vi "main.vi"() -> ()   [LabVIEW 2014]
uses:
  <vilib>/picture/3D Picture Control/Object/Create Object (drawable).vi
  <vilib>/picture/3D Picture Control/Object/Add Object (reference).vi
  <vilib>/Instr/_visa.llb/VISA Configure Serial Port (Instr).vi
  <vilib>/picture/3D Picture Control/NI_3D Picture Control.lvlib
panel:
  out "AcceZ":i32
  out "AcceY":i32
  out "加速度":cluster{dbl, dbl, dbl}(graph)
  out "AcceX":i32
  out "HEANDING":i32
  out "BANK":i32
  out "PITCH":i32
  in  "停止":bool
  in  "打开":bool caption="stop"
  in  "校验位：":u16(ring) items=["  无校验", "  奇校验", "  偶校验"]
  in  "波特率：":u16(ring)=11 items=["   300", "   600", "   1200", "   2400", "   4800   ", "   9600", "   19200", "   38400", "   43000", "   56000", "   57600", "   115200"]
  in  "通讯口：":u16(ring) items=["   com1", "   com2", "   com3", "   com4", "   com5"]
  out "姿态":cluster{dbl, dbl, dbl}(graph) caption="波形图表"
  in  "上下移动":dbl(slide) scale=-10.0..10.0
  in  "左右移动":dbl(slide) scale=-10.0..10.0
  in  "前后移动":dbl(slide) scale=-10.0..10.0
  in  "缩放":dbl(knob)=2.2771854734286614 scale=0.0..10.0
  out "三维图片":refnum<vi>(3d-picture)
  out "工作指示灯":bool
  # "----pxc"
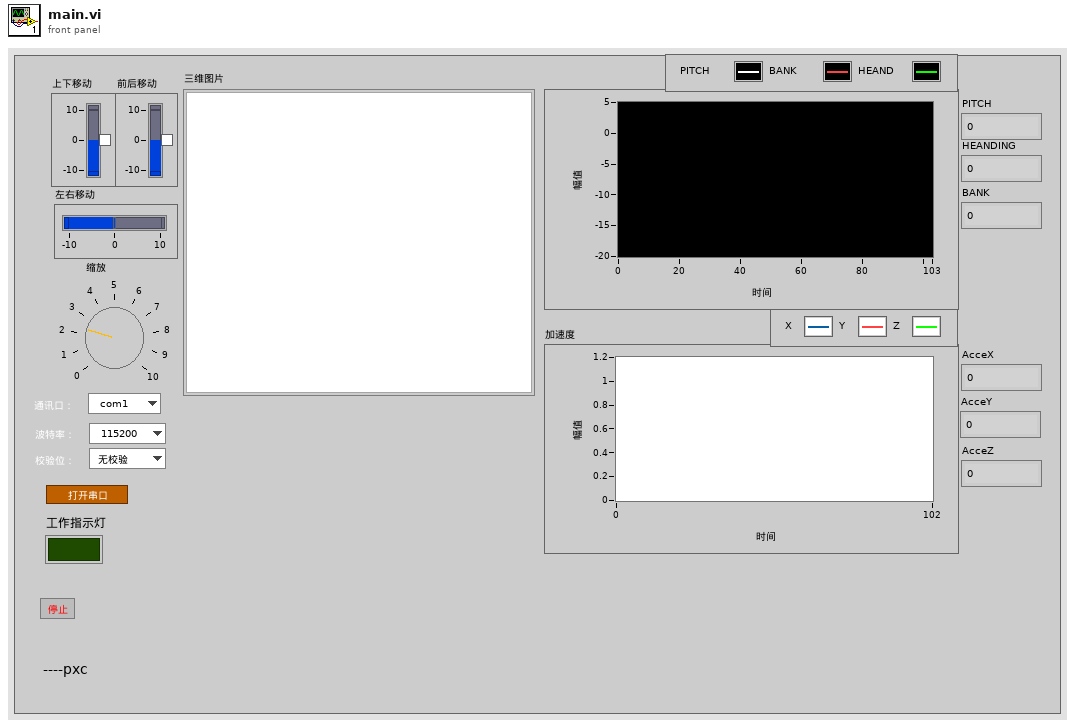
[diagram p1: front panel]
types:
  T1 = cluster{"PITCH":i32, "BANK":i32, "HEANDING":i32, "T":i32}
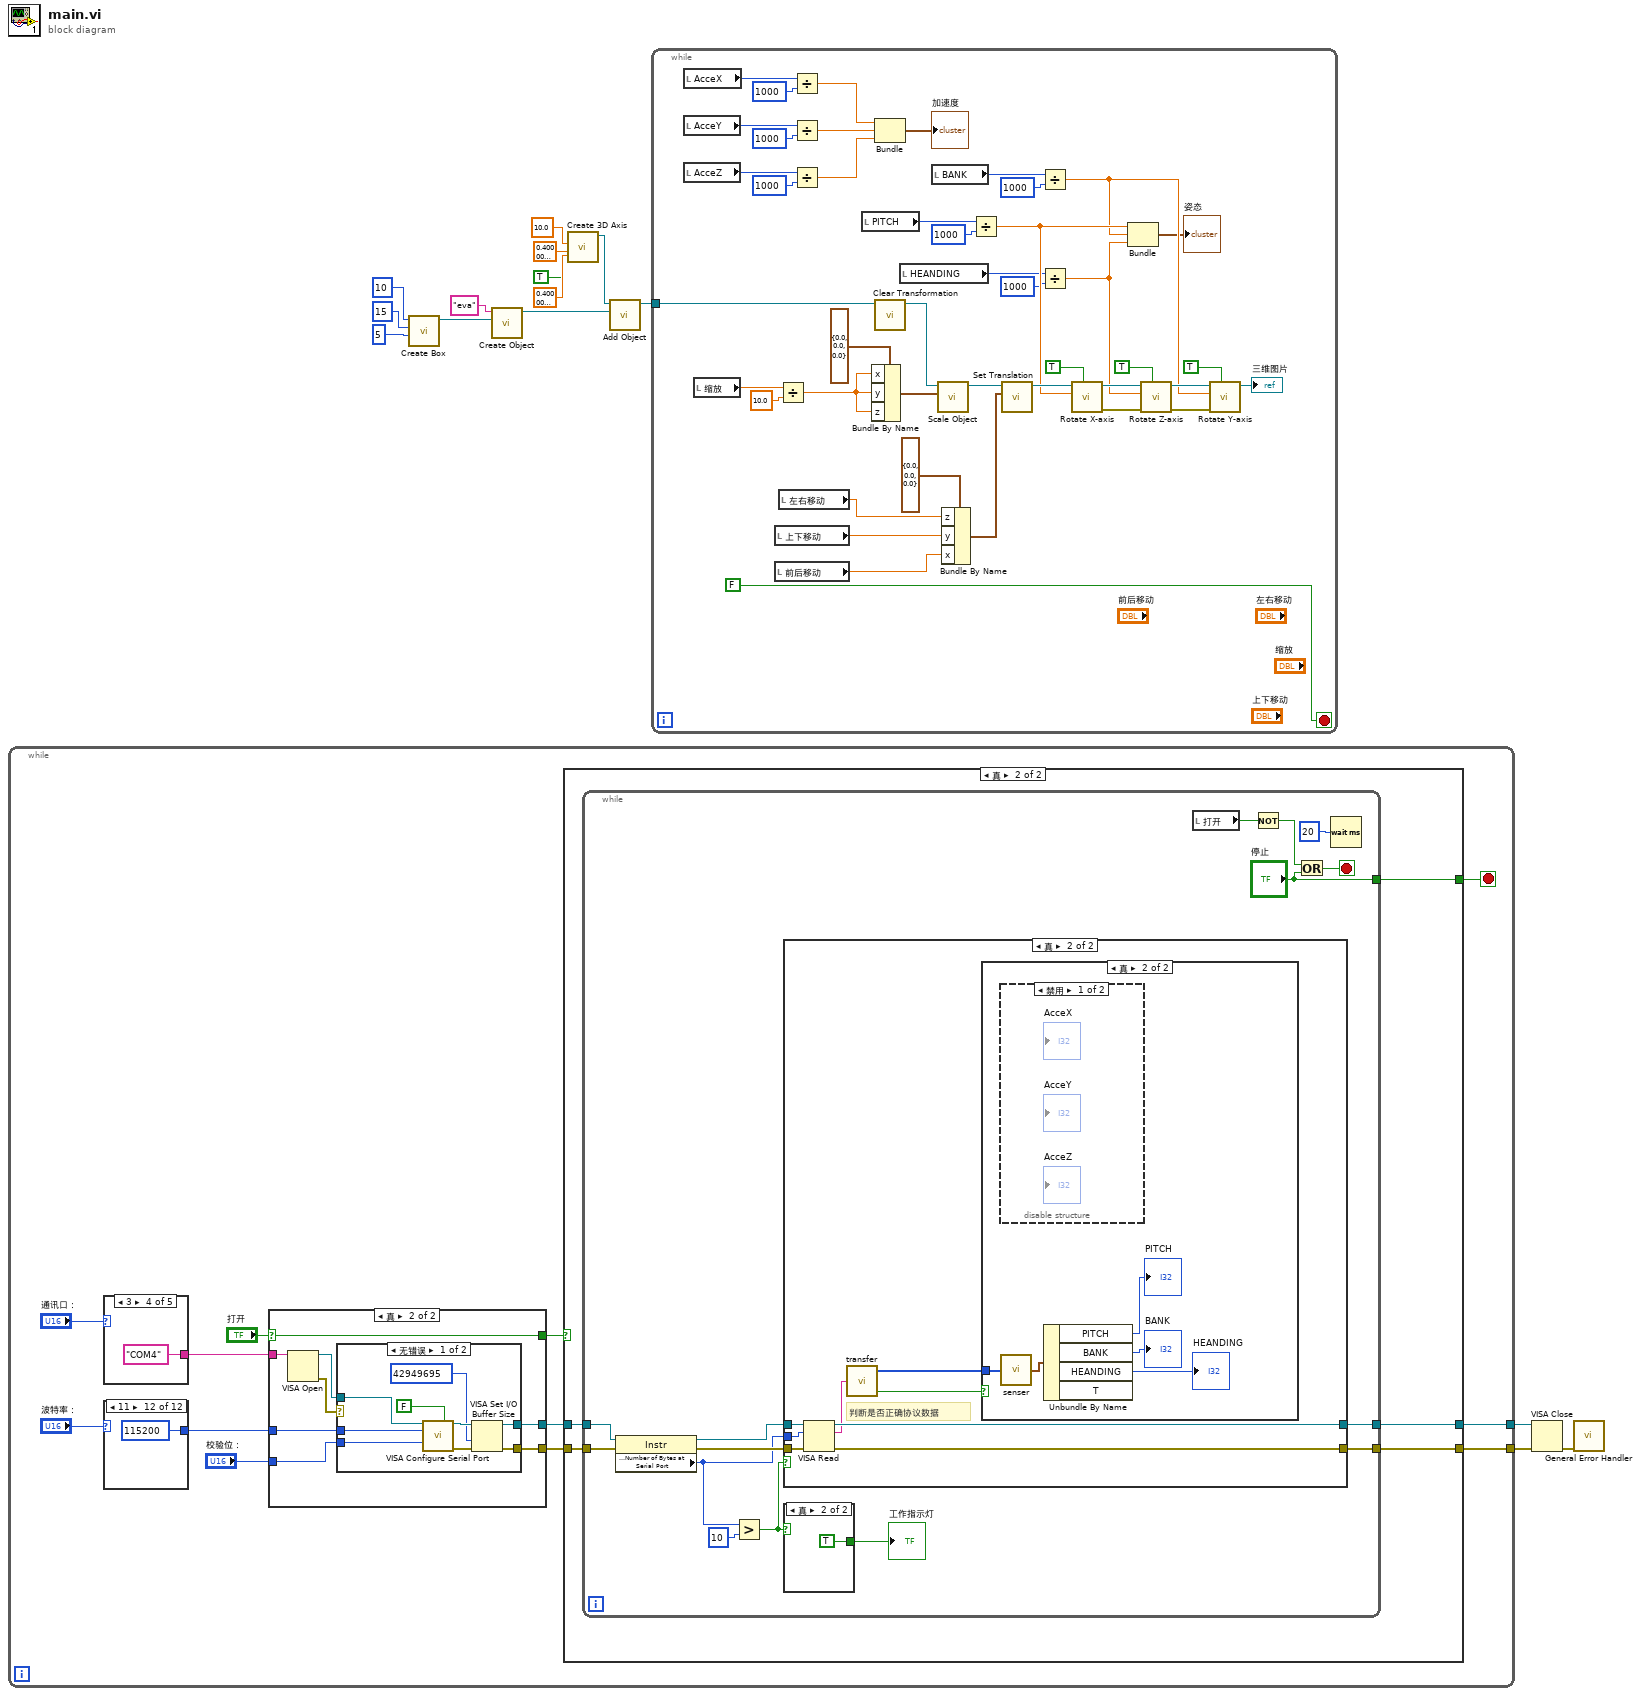
[diagram p0: block diagram]
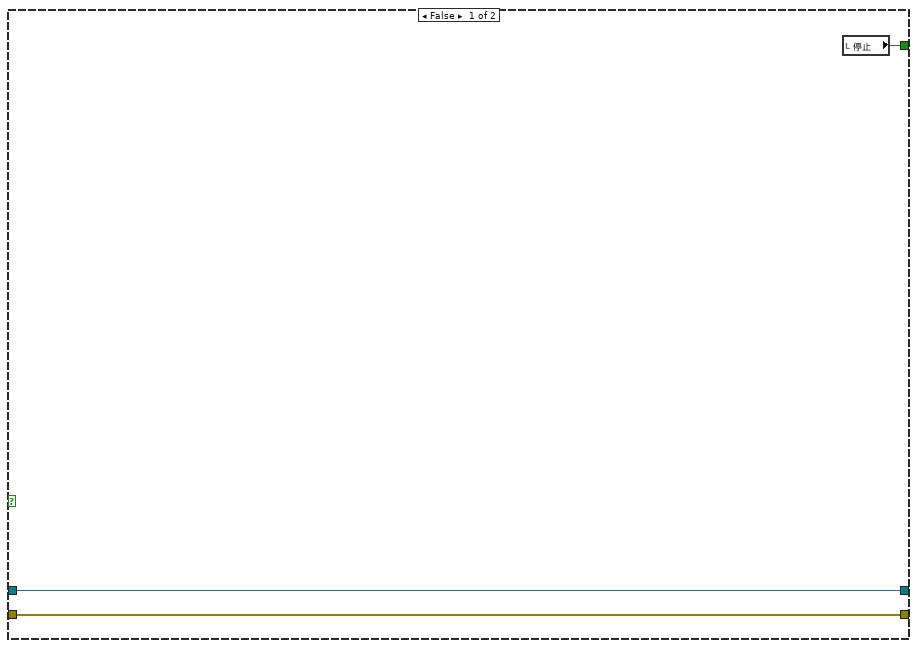
[diagram p2: hidden frame]
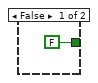
[diagram p6: hidden frame]
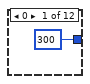
[diagram p7: hidden frame]
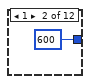
[diagram p8: hidden frame]
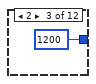
[diagram p9: hidden frame]
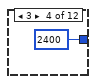
[diagram p10: hidden frame]
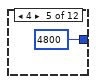
[diagram p11: hidden frame]
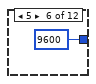
[diagram p12: hidden frame]
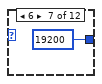
[diagram p13: hidden frame]
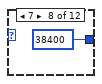
[diagram p14: hidden frame]
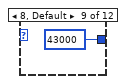
[diagram p15: hidden frame]
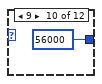
[diagram p16: hidden frame]
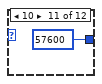
[diagram p17: hidden frame]
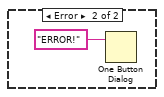
[diagram p19: hidden frame]
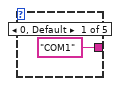
[diagram p20: hidden frame]
diagram:
  n1 = while {
    tunnel: [w26] -> w15
    tunnel: [w25] -> w14
    stop <- w17 stop-if-true
    n2 = case shown="3" "通讯口：" {
      tunnel: ["COM1" "COM2" "COM3" "COM4" "COM5"] -> w21
      frame 0, Default {
      }
      frame 1 {
      }
      frame 2 {
      }
      frame 3 {
      }
      frame 4 {
      }
    }
    n3 = case shown="11" "波特率：" {
      tunnel: [300 600 1200 2400 4800 9600 19200 38400 43000 56000 57600 115200] -> w18
      frame 0 {
      }
      frame 1 {
      }
      frame 2 {
      }
      frame 3 {
      }
      frame 4 {
      }
      frame 5 {
      }
      frame 6 {
      }
      frame 7 {
      }
      frame 8, Default {
      }
      frame 9 {
      }
      frame 10 {
      }
      frame 11 {
      }
    }
    n4 = case shown="真" "打开" {
      selector: "打开" -> [w80 w88]
      tunnel: w18 -> [_ w84]
      tunnel: [w80 w88] -> w16
      tunnel: [_ w82] -> w24
      tunnel: [_ w81] -> w27
      tunnel: w21 -> [_ w87]
      tunnel: "校验位：" -> [_ w83]
      frame False {
      }
      frame True {
        n5 = VISA Open(VISA resource name=w87) -> (VISA resource name=w85:refnum<visa-resource-name>, error out=w86:errorcluster)  [unwired: 4 in]
        n6 = case shown="无错误" w86 {
          tunnel: w85 -> [w97 _]
          tunnel: w84 -> [w96 _]
          tunnel: w83 -> [w95 _]
          tunnel: [w91 _] -> w82
          tunnel: [w92 _] -> w81
          frame No Error {
            n7 = call-poly "VISA Configure Serial Port"("VISA resource name"=w97, "Enable Termination\nChar (T)"=FALSE, "baud rate (9600)"=w96, "parity (0:none)"=w95) -> ("VISA resource name out"=w94:refnum<visa-resource-name>, "error out"=w93:errorcluster)  [unwired: 10 in]
            n8 = VISA Set I/O Buffer Size(VISA resource name=w94, size (4096)=u32 42949695 ("大小(4096)"), error in (no error)=w93) -> (VISA resource name out=w91:refnum<visa-resource-name>, error out=w92:errorcluster)  [unwired: 1 in]
          }
          frame Error {
            n9 = One Button Dialog(message="ERROR!" ("消息")) -> ()  [unwired: 1 in, 1 out]
          }
        }
      }
    }
    n10 = case shown="真" w16 {
      tunnel: w27 -> [w28 w35]
      tunnel: [w29 w34] -> w26
      tunnel: [w28 w33] -> w25
      tunnel: w24 -> [w29 w32]
      tunnel: [w30 w31] -> w17
      frame False {
        n11 = local read "停止"() -> (w30:bool)
      }
      frame True {
        n12 = while {
          tunnel: w32 -> [w42]
          tunnel: w35 -> [w41]
          tunnel: [w50] -> w34
          tunnel: [w49] -> w33
          tunnel: ["停止"] -> w31
          stop <- w46 stop-if-true
          n13 = property class="Instr"(reference=w42, error in=w41) -> (reference out=w39:refnum<visa-resource-name>, error out=w38:errorcluster, "Serial Settings:Number of Bytes at Serial Port"=w37:u32)
          n14 = Greater?(x=w37, y=u32 10) -> (0:w47:bool)
          n15 = case shown="真" w47 {
            tunnel: [w51 w54] -> w49
            tunnel: w39 -> [w52 w60]
            tunnel: w38 -> [w51 w55]
            tunnel: [w52 w59] -> w50
            tunnel: w37 -> [_ w58]
            frame False {
            }
            frame True {
              # "判断是否正确协议数据"
              n16 = VISA Read(VISA resource name=w60, byte count=w58, error in (no error)=w55) -> (VISA resource name out=w59:refnum<visa-resource-name>, read buffer=w57:string, error out=w54:errorcluster)  [unwired: 1 out]
              n17 = call "transfer.vi"("输入"=w57) -> ("待处理数据输出"=w56:u8[], "接收输出"=w53:bool)  [unwired: 1 out]
              n18 = case shown="真" w53 {
                tunnel: w56 -> [_ w65]
                frame False {
                }
                frame True {
                  n19 = disable-structure shown="禁用" {
                    frame Disabled {
                    }
                    frame Enabled {
                    }
                  }
                  n20 = call "senser.vi"("待处理数据"=w65) -> ("输出簇"=w64:T1)
                  n21 = Unbundle By Name(w64) -> ("PITCH"=→"PITCH":i32, "BANK"=→"BANK":i32, "HEANDING"=→"HEANDING":i32)  [unwired: 1 out]
                }
              }
            }
          }
          n22 = case shown="真" w47 {
            tunnel: [FALSE ("工作指示灯") TRUE ("工作指示灯")] -> w48
            frame False {
            }
            frame True {
            }
          }
          "工作指示灯" <- w48
          n23 = local read "打开"() -> (w44:bool)
          n24 = Not(x=w44) -> (.not. x?=w45:bool)
          n25 = Or(x=w45, y="停止") -> (x .or. y?=w46:bool)
          n26 = Wait (ms)(milliseconds to wait=u32 20 ("等待时间（毫秒）")) -> ()  [unwired: 1 out]
        }
      }
    }
  }
  n27 = call <vilib>:"Create Box.vi"("Length Z"=5, "Length Y"=15, "Length X"=10) -> ("New Box Refnum"=w6:refnum<vi>)  [unwired: 7 in, 1 out]
  n28 = call-poly <vilib>:"Create Object.vi"("Geometry"=w6, "Name"="eva") -> ("Scene:New Object"=w7:refnum<vi>)  [unwired: 8 in, 1 out]
  n29 = call <vilib>:"Create 3D Axis.vi"("Character Size"=sgl 0.4, "Axis label?"=TRUE, "Radius"=sgl 0.4, "Length"=sgl 10.0) -> ("New Object Refnum"=w12:refnum<vi>)  [unwired: 6 in, 1 out]
  n30 = call-poly <vilib>:"Add Object.vi"("New Object In"=w7, "Scene Object In"=w12) -> ("Scene Object Out"=w1:refnum<vi>)  [unwired: 7 in, 2 out]
  n31 = while {
    tunnel: w1 -> [w105]
    stop <- FALSE stop-if-true
    n32 = local read "AcceX"() -> (w115:i32)
    n33 = local read "AcceY"() -> (w113:i32)
    n34 = local read "AcceZ"() -> (w111:i32)
    n35 = local read "缩放"() -> (w138:dbl)
    n36 = local read "上下移动"() -> (w136:dbl)
    n37 = local read "前后移动"() -> (w135:dbl)
    n38 = Divide(x=w138, y=10.0) -> (x/y=w142:dbl)
    n39 = local read "左右移动"() -> (w137:dbl)
    n40 = Divide(x=w115, y=1000) -> (x/y=w109:dbl)
    n41 = Divide(x=w113, y=1000) -> (x/y=w108:dbl)
    n42 = Divide(x=w111, y=1000) -> (x/y=w107:dbl)
    n43 = local read "PITCH"() -> (w121:i32)
    n44 = Bundle By Name(cluster=cluster{"x":dbl, "y":dbl, "z":dbl} {"x"=0.0, "y"=0.0, "z"=0.0}, "x"=w142, "y"=w142, "z"=w142) -> (w144:cluster{"x":dbl, "y":dbl, "z":dbl})
    n45 = Bundle(w109, w108, w107) -> (→"加速度":cluster{dbl, dbl, dbl})  [unwired: 1 in]
    n46 = call <vilib>:"Clear Transformation.vi"("Object Refnum In"=w105) -> ("Object Refnum Out"=w146:refnum<vi>)  [unwired: 9 in, 1 out]
    n47 = local read "HEANDING"() -> (w117:i32)
    n48 = local read "BANK"() -> (w122:i32)
    n49 = call <vilib>:"Scale Object.vi"("Scale"=w144, "Scene.Object In"=w146) -> ("Scene.Object Out"=w145:refnum<vi>)  [unwired: 8 in, 1 out]
    n50 = Bundle By Name(cluster=cluster{"x":dbl, "y":dbl, "z":dbl} {"x"=0.0, "y"=0.0, "z"=0.0}, "z"=w137, "y"=w136, "x"=w135) -> (w141:cluster{"x":dbl, "y":dbl, "z":dbl})
    n51 = Divide(x=w121, y=1000) -> (x/y=w120:dbl)
    n52 = call <vilib>:"Set Translation.vi"("Translation"=w141, "Scene Object"=w145) -> ("Translated Object"=w132:refnum<vi>)  [unwired: 8 in, 1 out]
    n53 = Divide(x=w122, y=1000) -> (x/y=w119:dbl)
    n54 = Divide(x=w117, y=1000) -> (x/y=w123:dbl)
    n55 = call <vilib>:"Rotate X-axis.vi"("Relative?"=TRUE, "angle"=w120, "Scene Object In"=w132) -> ("error out"=w131:errorcluster, "Scene Object Out"=w130:refnum<vi>)  [unwired: 7 in]
    n56 = Bundle(w120, w119, w123) -> (→"姿态":cluster{dbl, dbl, dbl})  [unwired: 1 in]
    n57 = call <vilib>:"Rotate Z-axis.vi"("Relative?"=TRUE, "error in (no error)"=w131, "angle"=w123, "Scene Object In"=w130) -> ("error out"=w127:errorcluster, "Scene Object Out"=w126:refnum<vi>)  [unwired: 6 in]
    n58 = call <vilib>:"Rotate Y-axis.vi"("Relative?"=TRUE, "error in (no error)"=w127, "angle"=w119, "Scene Object In"=w126) -> ("Scene Object Out"=→"三维图片":refnum<vi>)  [unwired: 6 in, 1 out]
  }
  n59 = VISA Close(VISA resource name=w15, error in (no error)=w14) -> (error out=w13:errorcluster)
  n60 = call <vilib>:"General Error Handler.vi"("error in (no error)"=w13) -> ()  [unwired: 10 in, 5 out]
